vi "FeedbackDecode_RmDEKAThresh.vi"(2 "ValIn":dbl, 3 "Thresh":dbl min=0.0 max=1.0) -> (0 "ValOut":dbl)   [LabVIEW 2020]
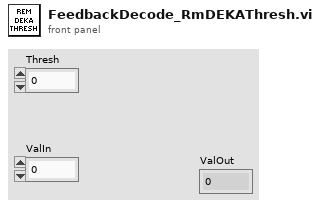
[diagram p1: front panel]
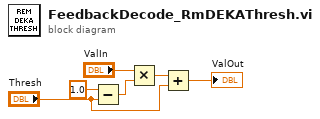
[diagram p0: block diagram]
diagram:
  n1 = Subtract(x=1.0, y="Thresh") -> (x-y=w5:dbl)
  n2 = Multiply(x="ValIn", y=w5) -> (x*y=w6:dbl)
  n3 = Add(x=w6, y="Thresh") -> (x+y=→"ValOut":dbl)
